vi "main-20220123.vi"() -> ()   [LabVIEW 2019]
panel:
  out "error out":errorcluster
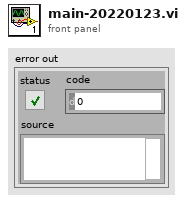
[diagram p1: front panel]
types:
  T1 = enum16{"right", "left", "up", "down", "rightup", "rightdown", "leftup", "leftdown"}[]
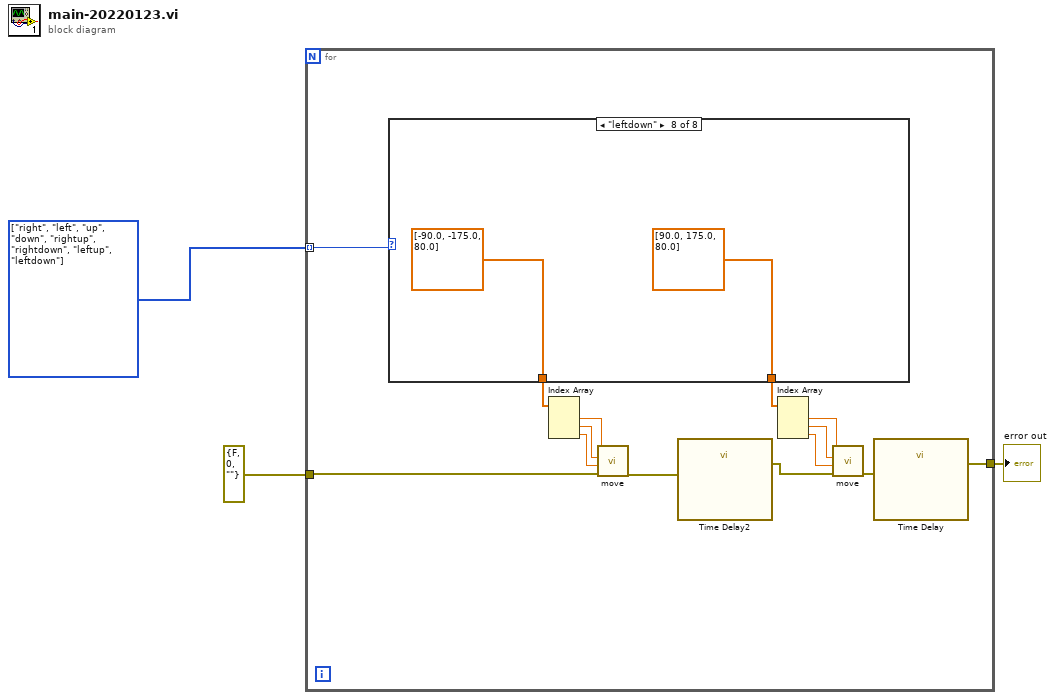
[diagram p0: block diagram]
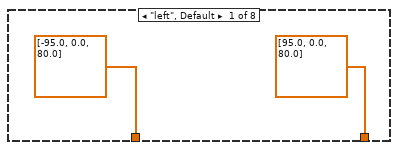
[diagram p2: hidden frame]
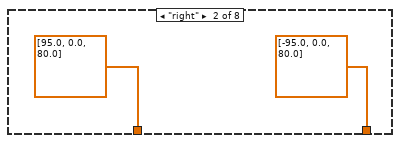
[diagram p3: hidden frame]
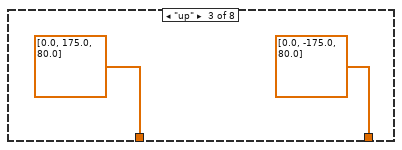
[diagram p4: hidden frame]
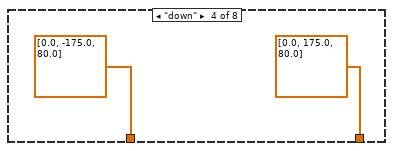
[diagram p5: hidden frame]
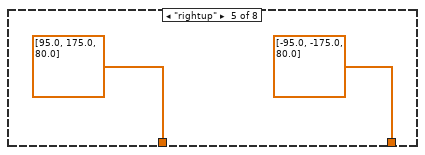
[diagram p6: hidden frame]
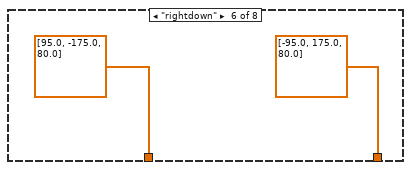
[diagram p7: hidden frame]
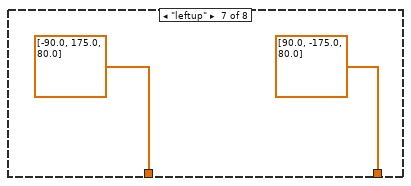
[diagram p8: hidden frame]
diagram:
  w2 = T1 [enum."right", enum."left", enum."up", enum."down", enum."rightup", enum."rightdown", enum."leftup", enum."leftdown"] items=["right", "left", "up", "down", "rightup", "rightdown", "leftup", "leftdown"]
  n1 = for {
    tunnel: [w16] -> w1
    tunnel: errorcluster {"status"=FALSE, "code"=0, "source"=""} ("error constant") -> [w13]
    tunnel: w2 -> [w4] mode=indexing
    n2 = case shown="\"leftdown\"" w4 {
      tunnel: [dbl[] [95.0, 0.0, 80.0] dbl[] [-95.0, 0.0, 80.0] dbl[] [0.0, -175.0, 80.0] dbl[] [0.0, 175.0, 80.0] dbl[] [-95.0, -175.0, 80.0] dbl[] [-95.0, 175.0, 80.0] dbl[] [90.0, -175.0, 80.0] dbl[] [90.0, 175.0, 80.0]] -> w6
      tunnel: [dbl[] [-95.0, 0.0, 80.0] dbl[] [95.0, 0.0, 80.0] dbl[] [0.0, 175.0, 80.0] dbl[] [0.0, -175.0, 80.0] dbl[] [95.0, 175.0, 80.0] dbl[] [95.0, -175.0, 80.0] dbl[] [-90.0, 175.0, 80.0] dbl[] [-90.0, -175.0, 80.0]] -> w5
      frame "left", Default {
      }
      frame "right" {
      }
      frame "up" {
      }
      frame "down" {
      }
      frame "rightup" {
      }
      frame "rightdown" {
      }
      frame "leftup" {
      }
      frame "leftdown" {
      }
    }
    n3 = Index Array(array=w5) -> (element #1=w7:dbl, element #2=w8:dbl, element #3=w9:dbl)  [unwired: 3 in]
    n4 = call "move.vi"("error in (no error)"=w13, "RPM"=w9, "y"=w8, "X"=w7) -> ("error out"=w14:errorcluster)  [unwired: 7 in]
    n5 = call "Time Delay2"("error in (no error)"=w14) -> ("error out"=w15:errorcluster)  [unwired: 10 in]
    n6 = Index Array(array=w6) -> (element #1=w10:dbl, element #2=w11:dbl, element #3=w12:dbl)  [unwired: 3 in]
    n7 = call "move.vi"("error in (no error)"=w15, "RPM"=w12, "y"=w11, "X"=w10) -> ("error out"=w17:errorcluster)  [unwired: 7 in]
    n8 = call "Time Delay"("error in (no error)"=w17) -> ("error out"=w16:errorcluster)  [unwired: 10 in]
  }
  "error out" <- w1
